vi "CreateStreamFilePath.vi"(8 "error in (no error)":errorcluster, 9 "data group":string, 10 "block":i32, 11 "stream id":string) -> (0 "error out":errorcluster, 3 "file path":path)   [LabVIEW 2017, in "FileManager.lvlib"]
uses:
  <vilib>/addons/InsightCM/Devices/Shared/Common/FileManager/FileManager.lvlib
  <vilib>/addons/InsightCM/Utilities/GlobalConfiguration/GlobalConfiguration.lvlib
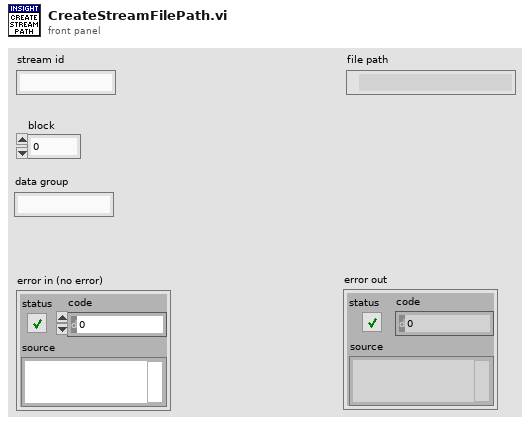
[diagram p1: front panel]
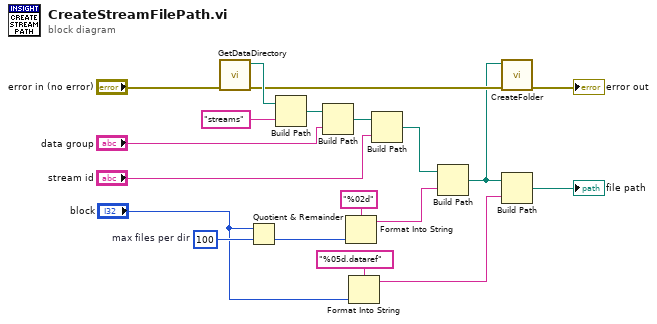
[diagram p0: block diagram]
diagram:
  w12 = 100  # max files per dir
  n1 = call <vilib>:"GetDataDirectory.vi"("error in (no error)"="error in (no error)") -> ("error out"=w16:errorcluster, "data directory"=w18:path)  [unwired: 9 in]
  n2 = Quotient & Remainder(x="block", y=w12) -> (floor(x/y)=w9:i32)  [unwired: 1 out]
  n3 = Build Path(base path=w18, name or relative path="streams") -> (appended path=w2:path)
  n4 = Build Path(base path=w2, name or relative path="data group") -> (appended path=w1:path)
  n5 = Format Into String(format string="%02d", w9) -> (resulting string=w8:string)  [unwired: 2 in, 1 out]
  n6 = Format Into String(format string="%05d.dataref", "block") -> (resulting string=w5:string)  [unwired: 2 in, 1 out]
  n7 = Build Path(base path=w1, name or relative path="stream id") -> (appended path=w11:path)
  n8 = Build Path(base path=w11, name or relative path=w8) -> (appended path=w7:path)
  n9 = call <vilib>:"CreateFolder.vi"("error in (no error)"=w16, "folder"=w7) -> ("error out"=→"error out":errorcluster)  [unwired: 8 in, 1 out]
  n10 = Build Path(base path=w7, name or relative path=w5) -> (appended path=→"file path":path)
